vi "Parse (Acceleration, Angular Rate, And Magnetometer Vectors).vi"(7 "Message In":string) -> (6 "Magnetometer Vector":sgl[](array[numeric]), 8 "Acceleration":sgl[](array[numeric]), 10 "Angular Rate":sgl[](array[numeric]), 15 "Timer":u32)   [LabVIEW 2012, in "MicroStrain 3DM-GXx.lvlib"]
doc: "Parse the data from the 0xCB message into an Acceleration Vector (m/s^2), an Angular Rate Vector (rad/s) and a Magnetometer Vector (G)."
uses:
  <instrlib>/MicroStrain 3DM-GXx/MicroStrain 3DM-GXx.lvlib
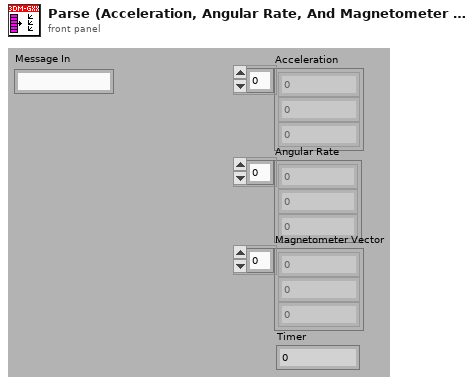
[diagram p1: front panel]
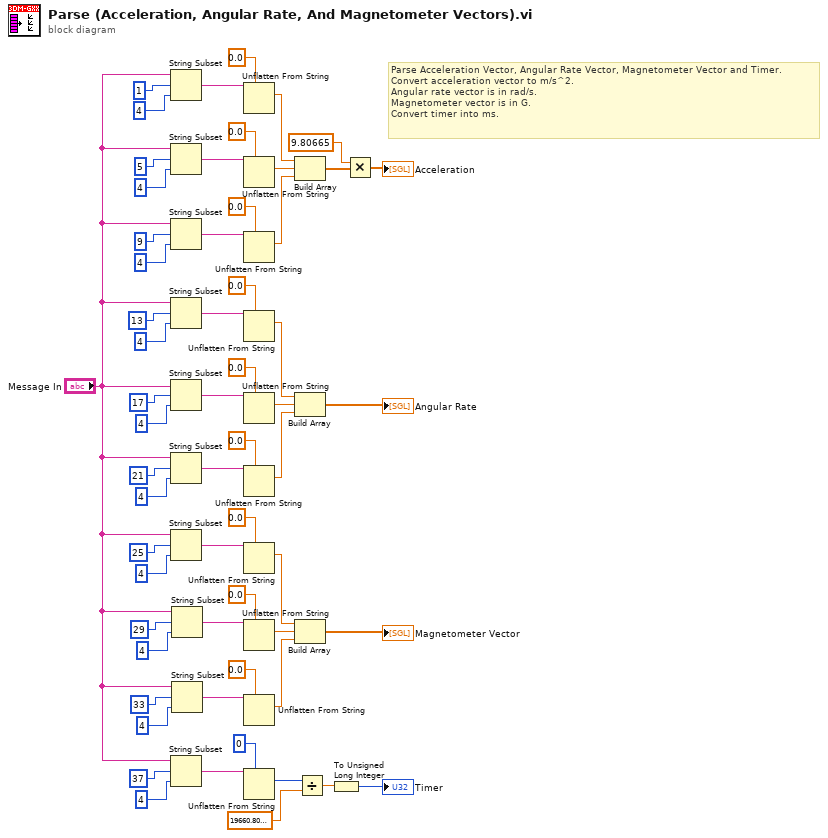
[diagram p0: block diagram]
diagram:
  # "Parse Acceleration Vector, Angular Rate Vector, Magnetometer Vector and Timer.\nConvert acceleration vector to m/s^2.\nAngular rate vector is in rad/s.\nMagnetometer vector is in G.\nConvert timer into ms."
  n1 = String Subset(string="Message In", offset (0)=1, length (rest)=4 ("length (rest)")) -> (substring=w57:string)
  n2 = String Subset(string="Message In", offset (0)=5, length (rest)=4 ("length (rest)")) -> (substring=w54:string)
  n3 = String Subset(string="Message In", offset (0)=9, length (rest)=4 ("length (rest)")) -> (substring=w49:string)
  n4 = String Subset(string="Message In", offset (0)=13, length (rest)=4 ("length (rest)")) -> (substring=w46:string)
  n5 = String Subset(string="Message In", offset (0)=17, length (rest)=4 ("length (rest)")) -> (substring=w41:string)
  n6 = String Subset(string="Message In", offset (0)=21, length (rest)=4 ("length (rest)")) -> (substring=w38:string)
  n7 = String Subset(string="Message In", offset (0)=25, length (rest)=4 ("length (rest)")) -> (substring=w33:string)
  n8 = String Subset(string="Message In", offset (0)=37, length (rest)=4 ("length (rest)")) -> (substring=w22:string)
  n9 = String Subset(string="Message In", offset (0)=29, length (rest)=4 ("length (rest)")) -> (substring=w30:string)
  n10 = String Subset(string="Message In", offset (0)=33, length (rest)=4 ("length (rest)")) -> (substring=w25:string)
  n11 = Unflatten From String(type=sgl 0.0, binary string=w57) -> (value=w16:sgl)  [unwired: 3 in, 2 out]
  n12 = Unflatten From String(type=sgl 0.0, binary string=w54) -> (value=w17:sgl)  [unwired: 3 in, 2 out]
  n13 = Unflatten From String(type=sgl 0.0, binary string=w49) -> (value=w15:sgl)  [unwired: 3 in, 2 out]
  n14 = Unflatten From String(type=sgl 0.0, binary string=w46) -> (value=w14:sgl)  [unwired: 3 in, 2 out]
  n15 = Unflatten From String(type=sgl 0.0, binary string=w41) -> (value=w13:sgl)  [unwired: 3 in, 2 out]
  n16 = Unflatten From String(type=sgl 0.0, binary string=w38) -> (value=w12:sgl)  [unwired: 3 in, 2 out]
  n17 = Unflatten From String(type=sgl 0.0, binary string=w33) -> (value=w9:sgl)  [unwired: 3 in, 2 out]
  n18 = Unflatten From String(type=sgl 0.0, binary string=w30) -> (value=w10:sgl)  [unwired: 3 in, 2 out]
  n19 = Unflatten From String(type=sgl 0.0, binary string=w25) -> (value=w8:sgl)  [unwired: 3 in, 2 out]
  n20 = Unflatten From String(type=u32 0, binary string=w22) -> (value=w6:u32)  [unwired: 3 in, 2 out]
  n21 = Build Array(w16, w17, w15) -> (w4:sgl[])
  n22 = Build Array(w14, w13, w12) -> (→"Angular Rate":sgl[])
  n23 = Build Array(w9, w10, w8) -> (→"Magnetometer Vector":sgl[])
  n24 = Divide(x=w6, y=sgl 19660.8) -> (x/y=w2:sgl)
  n25 = To Unsigned Long Integer(number=w2) -> (unsigned 32bit integer=→"Timer":u32)
  n26 = Multiply(x=9.80665, y=w4) -> (x*y=→"Acceleration":dbl[])
